vi "RnachT.vi"(1 "AVS Channel":u16(ring) items=["Ch3"=3, "Ch5"=5, "Ch6"=6, "Ch7"=7], 2 "R":dbl=11430.0 format="%.2f", 3 "Sensor Cal#":u16(ring) items=["no calibration", "leer", "U02453 Dryo", "U03411 Mischer", "U04184 JT", "alt", "1D Lin Interpol"]) -> (0 "T (K)":dbl=0.00957168277075326 format="%^.3e")   [LabVIEW 2018]
uses:
  Instrument_Setup.vi
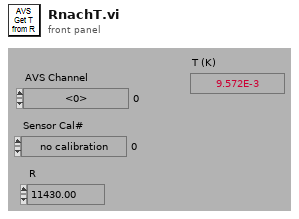
[diagram p1: front panel]
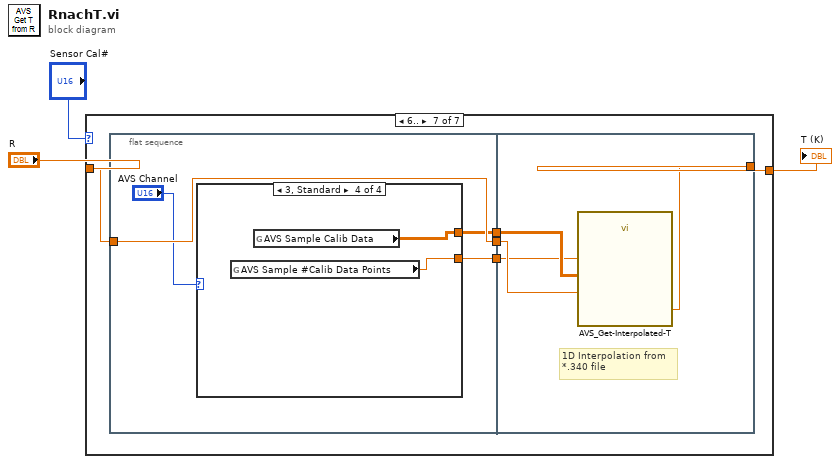
[diagram p0: block diagram]
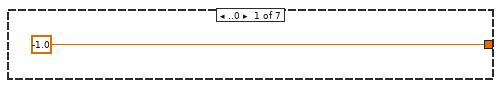
[diagram p2: hidden frame]
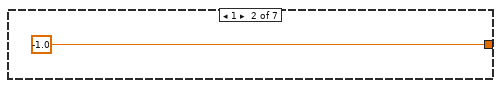
[diagram p3: hidden frame]
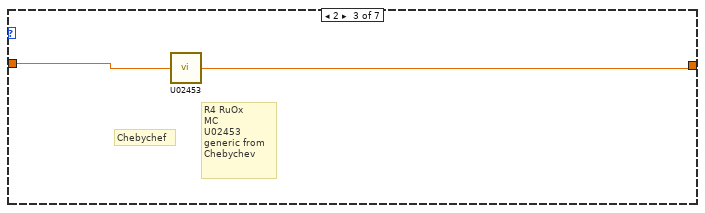
[diagram p4: hidden frame]
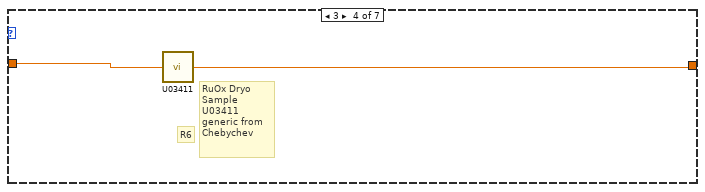
[diagram p5: hidden frame]
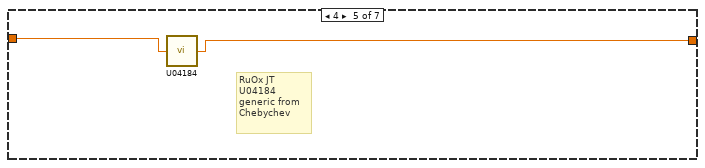
[diagram p6: hidden frame]
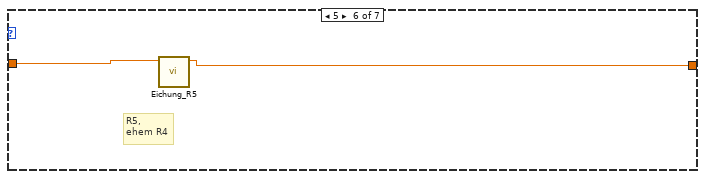
[diagram p7: hidden frame]
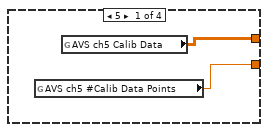
[diagram p8: hidden frame]
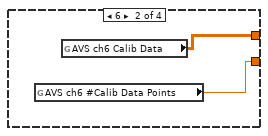
[diagram p9: hidden frame]
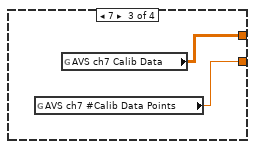
[diagram p10: hidden frame]
diagram:
  n1 = case shown="6.." "Sensor Cal#" {
    tunnel: "R" -> [_ _ w7 w9 w11 w12 w18]
    tunnel: [-1.0 ("T (K)") -1.0 ("T (K)") w6 w8 w10 w13 w17] -> w2
    frame ..0 {
    }
    frame 1 {
    }
    frame 2 {
      # "R4 RuOx\nMC\nU02453\ngeneric from \nChebychev"
      # "Chebychef"
      n2 = call "U02453.vi"("R (Ohm)"=w7) -> ("T (K)"=w6:dbl)
    }
    frame 3 {
      # "RuOx Dryo\nSample\nU03411\ngeneric from \nChebychev"
      # "R6"
      n3 = call "U03411.vi"("R (Ohm)"=w9) -> ("T (K)"=w8:dbl)
    }
    frame 4 {
      # "RuOx JT\nU04184\ngeneric from \nChebychev"
      n4 = call "U04184.vi"("R (Ohm)"=w11) -> ("T (K)"=w10:dbl)
    }
    frame 5 {
      # "R5,\nehem R4"
      n5 = call "Eichung_R5.vi"("R (Ohm)"=w12) -> ("T (K)"=w13:dbl)  [unwired: 10 in]
    }
    frame 6.. {
      n6 = flat-sequence {
        tunnel: w18 -> [w22]
        tunnel: [w22] -> w16
        tunnel: [w20] -> w15
        tunnel: [w19] -> w14
        tunnel: [w33] -> w17
        tunnel: w16 -> [w34]
        tunnel: w15 -> [w32]
        tunnel: w14 -> [w31]
        frame #0 {
          n7 = case shown="3, Standard" "AVS Channel" {
            tunnel: [w24 w26 w28 w30] -> w20
            tunnel: [w23 w25 w27 w29] -> w19
            frame 5 {
              n8 = global read "Instrument_Setup.vi" "AVS ch5 #Calib Data Points"() -> (w23:dbl)
              n9 = global read "Instrument_Setup.vi" "AVS ch5 Calib Data"() -> (w24:dbl[][])
            }
            frame 6 {
              n10 = global read "Instrument_Setup.vi" "AVS ch6 #Calib Data Points"() -> (w25:dbl)
              n11 = global read "Instrument_Setup.vi" "AVS ch6 Calib Data"() -> (w26:dbl[][])
            }
            frame 7 {
              n12 = global read "Instrument_Setup.vi" "AVS ch7 #Calib Data Points"() -> (w27:dbl)
              n13 = global read "Instrument_Setup.vi" "AVS ch7 Calib Data"() -> (w28:dbl[][])
            }
            frame 3, Default {
              n14 = global read "Instrument_Setup.vi" "AVS Sample #Calib Data Points"() -> (w29:dbl)
              n15 = global read "Instrument_Setup.vi" "AVS Sample Calib Data"() -> (w30:dbl[][])
            }
          }
        }
        frame #1 {
          # "1D Interpolation from\n*.340 file"
          n16 = call "AVS_Get-Interpolated-T.vi"("# of Data Points"=w31, "Calibration Datapoints"=w32, "Resistance value"=w34) -> ("Interpolated Termperature scalar"=w33:dbl)  [unwired: 8 in]
        }
      }
    }
  }
  "T (K)" <- w2
